vi "Resize 2D array.vi"(4 "Maintain Aspect ratio? (T)":bool=TRUE, 5 "New Width":i32, 6 "New Height":i32, 7 "2D Array In":u32[][](array[numeric])) -> (2 "new picture":picture, 3 "Resized Array":u32[][](array[numeric]))   [LabVIEW 2011]
uses:
  <vilib>/picture/picture.llb/Draw True-Color Pixmap.vi
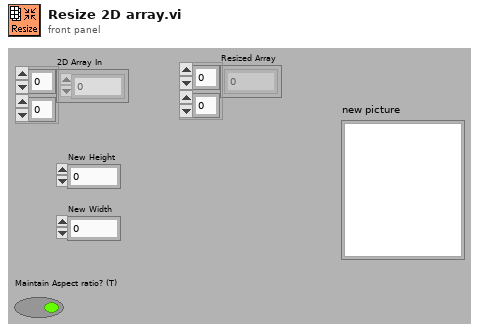
[diagram p1: front panel]
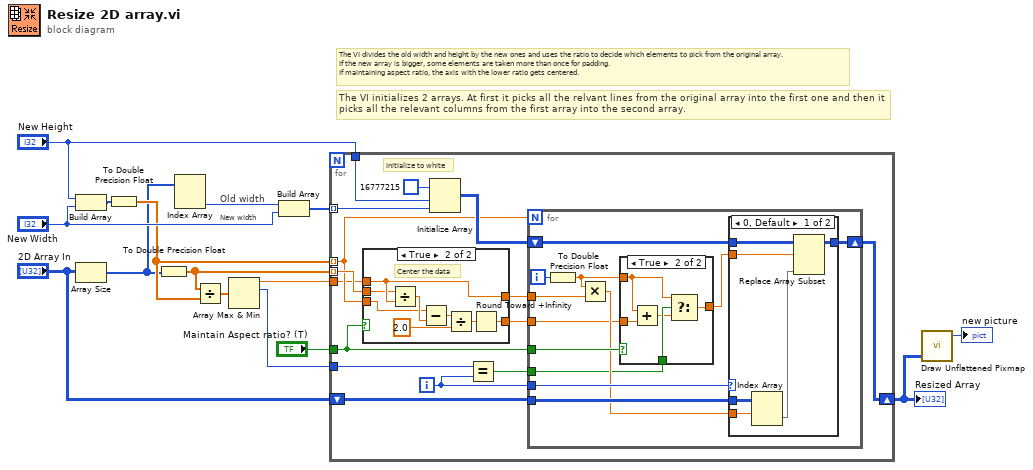
[diagram p0: block diagram]
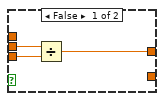
[diagram p2: hidden frame]
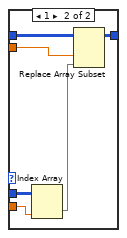
[diagram p4: hidden frame]
diagram:
  # "New width"
  # "The VI initializes 2 arrays. At first it picks all the relvant lines from the original array into the first one and then it picks all the relevant columns from the first array into the second array."
  # "The VI divides the old width and height by the new ones and uses the ratio to decide which elements to pick from the original array.\nIf the new array is bigger, some elements are taken more than once for padding. \nIf maintaining aspect ratio, the axis with the lower ratio gets centered."
  # "Old width"
  n1 = Build Array("New Height", "New Width") -> (w7:i32[])
  n2 = Array Size(array="2D Array In") -> (size(s)=w1:i32[])
  n3 = To Double Precision Float(number=w7) -> (double precision float=w3:dbl[])
  n4 = To Double Precision Float(number=w1) -> (double precision float=w2:dbl[])
  n5 = Index Array(array=w1) -> (element #2=w15:i32)  [unwired: 2 in, 1 out]
  n6 = Divide(x=w2, y=w3) -> (x/y=w13:dbl[])
  n7 = Array Max & Min(array=w13) -> (max value=w6:dbl, max index (indices)=w4:i32)  [unwired: 2 out]
  n8 = Build Array(w15, "New Width") -> (w8:i32[])
  n9 = for {
    tunnel: w2 -> [w25] mode=indexing
    tunnel: w3 -> [w23] mode=indexing
    shift-right: [w30] -> w12
    shift-left: "2D Array In" -> [w29]
    tunnel: "New Height" -> [w27]
    tunnel: w8 -> [w26] mode=indexing
    tunnel: w6 -> [w22]
    tunnel: "Maintain Aspect ratio? (T)" -> [w17]
    tunnel: w4 -> [w19]
    i -> [w20]
    # "Initialize to white"
    n10 = case shown="True" w17 {
      tunnel: w25 -> [w33 w35]
      tunnel: [w32 w41] -> w24
      tunnel: w23 -> [w31 w34]
      tunnel: w22 -> [_ w41]
      tunnel: [_ w36] -> w21
      frame False {
        n11 = Divide(x=w33, y=w31) -> (x/y=w32:dbl)
      }
      frame True {
        # "Center the data"
        n12 = Divide(x=w35, y=w41) -> (x/y=w37:dbl)
        n13 = Subtract(x=w34, y=w37) -> (x-y=w38:dbl)
        n14 = Divide(x=w38, y=2.0) -> (x/y=w40:dbl)
        n15 = Round Toward +Infinity(x=w40) -> (ceil(x): smallest int >= x=w36:dbl)
      }
    }
    n16 = Initialize Array(u32 16777215, w27, w26) -> (w28:u32[][])
    n17 = Equal?(x=w19, y=w20) -> (x = y?=w18:bool)
    n18 = for {
      N: w23 -> [_]
      tunnel: w24 -> [w53]
      tunnel: w29 -> [w52]
      shift-right: [w49] -> w30
      shift-left: w28 -> [w50]
      tunnel: w20 -> [w51]
      tunnel: w17 -> [w48]
      tunnel: w21 -> [w43]
      tunnel: w18 -> [w44]
      i -> [w45]
      n19 = To Double Precision Float(number=w45) -> (double precision float=w42:dbl)
      n20 = Multiply(x=w42, y=w53) -> (x*y=w47:dbl)
      n21 = case shown="True" w48 {
        tunnel: [w54 w59] -> w46
        tunnel: w42 -> [w54 w57]
        tunnel: w44 -> [_ w58]
        tunnel: w43 -> [_ w55]
        frame False {
        }
        frame True {
          n22 = Add(x=w57, y=w55) -> (x+y=w56:dbl)
          n23 = Select(t=w57, s=w58, f=w56) -> (s? t:f=w59:dbl)
        }
      }
      n24 = case shown="0, Default" w51 {
        tunnel: w52 -> [w65 w71]
        tunnel: w47 -> [w61 w67]
        tunnel: w50 -> [w64 w70]
        tunnel: [w63 w69] -> w49
        tunnel: w46 -> [w60 w66]
        frame 0, Default {
          n25 = Index Array(array=w65, index (row)=w61) -> (element=w62:u32[])  [unwired: 1 in]
          n26 = Replace Array Subset(array=w64, new element=w62, index (row)=w60) -> (w63:u32[][])  [unwired: 1 in]
        }
        frame 1 {
          n27 = Index Array(array=w71, index (col)=w67) -> (element=w68:u32[])  [unwired: 1 in]
          n28 = Replace Array Subset(array=w70, new element=w68, index (col)=w66) -> (w69:u32[][])  [unwired: 1 in]
        }
      }
    }
  }
  "Resized Array" <- w12
  n29 = call-poly <vilib>:"Draw Unflattened Pixmap.vi"("data (RGB format)"=w12) -> ("new picture"=→"new picture":picture)  [unwired: 8 in]
